vi "FUG_PowerSupply.destructor.vi"(0 "i ref in":refnum<vi>, 5 "error in(no error)":errorcluster) -> (19 "error out":errorcluster)   [LabVIEW 2014, in "FUG_PowerSupply.lvlib"]
doc: "This is the destructor of a class.\n\nLicense Agreement for this software:\n\nCopyright (C)\nGesellschaft für Schwerionenforschung, GSI\nPlanckstr. 1\n64291 Darmstadt\nGermany\n\nContact: D.Beck@gsi.de \n\nThis program is free software; you can redistribute it and/or modify it under the terms of the \nGNU General Public License as published by the Free Software Foundation; either version 2 of \nthe license, or (at your option) any later version.\n\nThis program is distributed in the hope that it will be useful, but WITHOUT ANY WARRANTY; \nwithout even the implied warranty of MERCHANTABILITY or FITNESS FOR A PARTICULAR PURPOSE. See the GNU General License for more details (http://www.gnu.org).\n\nGesellschaft für Schwerionenforschung, GSI\nPlanckstr. 1, 64291 Darmstadt, Germany\nFor all questions and ideas contact: M.Richter@gsi.de, H.Brand@gsi.de or D.Beck@gsi.de.\nLast update: 16-JUN-2004"
uses:
  FUG_PowerSupply.lvlib
  CS_Core/CSApplicationBaseClasses/PSChannelBase/PSChannelBase.lvlib
  CSlibraries-extern/DimLVEvent/LVDimInterface/LVDimInterface.lvlib
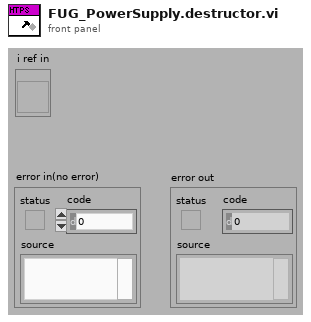
[diagram p1: front panel]
types:
  T1 = typedef "FUG_PowerSupply.lvlib/FUG_PowerSupply.i attribute.ctl" = cluster{"Type":string, "Elektrode Name":string, "CALC_FACTOR_SET_VOLTAGE":dbl, "CALC_FACTOR_GET_VOLTAGE":dbl, "CALC_FACTOR_GET_CURRENT":dbl, "CALC_FACTOR_SET_CURRENT ":dbl, "REG_VALUE":dbl, "Sign":bool, "setVoltID":i32, "setCurrentID":i32, "setPowerOnID":i32, "MaxVoltage":dbl}
  T2 = enum16{"SetAttribute", "GetAttribute", "CreateAttribute", "DestroyAttribute", "DestroyAllAtributes"}
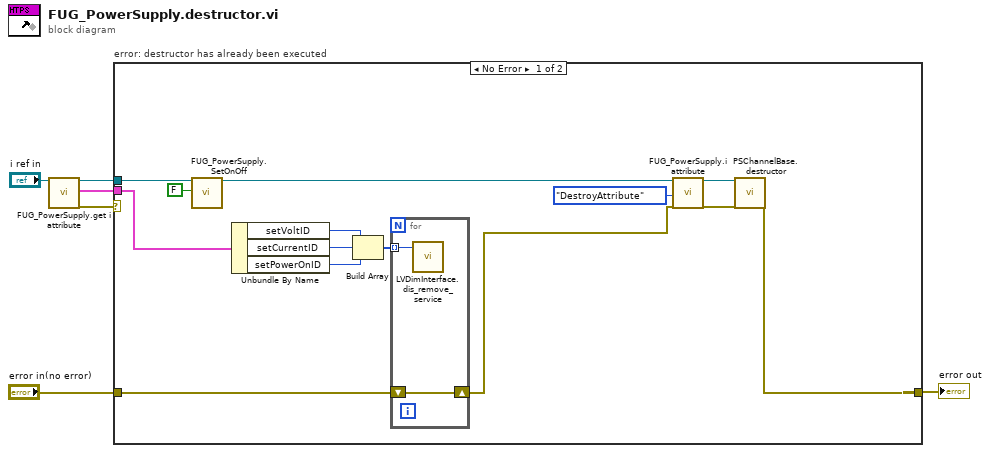
[diagram p0: block diagram]
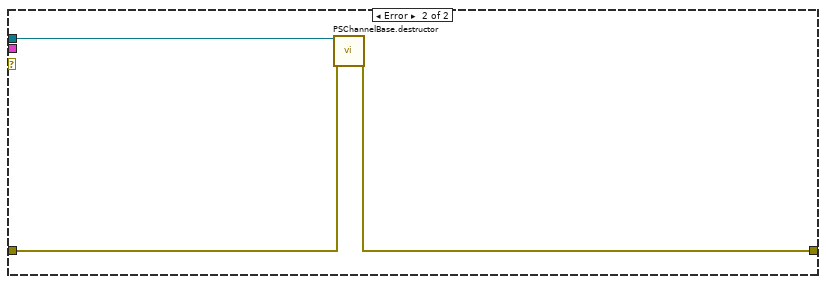
[diagram p2: hidden frame]
diagram:
  n1 = call "FUG_PowerSupply.get i attribute.vi"("i ref in"="i ref in") -> ("i ref out"=w5:refnum<vi>, "i attribute"=w4:T1, "error out"=w3:errorcluster)  [unwired: 16 in]
  n2 = case "error: destructor has already been executed" shown="No Error" w3 {
    tunnel: [w17 w23] -> w1
    tunnel: "error in(no error)" -> [w11 w24]
    tunnel: w5 -> [w9 w25]
    tunnel: w4 -> [w16 _]
    frame No Error {
      n3 = call "FUG_PowerSupply.SetOnOff.vi"("i ref in"=w9, "value"=FALSE) -> ("i ref out"=w8:refnum<vi>)  [unwired: 16 in, 1 out]
      n4 = Unbundle By Name(w16) -> ("setVoltID"=w14:i32, "setCurrentID"=w13:i32, "setPowerOnID"=w15:i32)
      n5 = Build Array(w14, w13, w15) -> (w12:i32[])
      n6 = for {
        tunnel: w12 -> [w22] mode=indexing
        shift-right: [w21] -> w10
        shift-left: w11 -> [w21]
        n7 = call "LVDimInterface.dis_remove_service.vi"("my_serviceID"=w22) -> ()  [unwired: 18 in, 1 out]
      }
      n8 = call "FUG_PowerSupply.i attribute.vi"("VI Refnum"=w8, "Action"=T2."DestroyAttribute", "error in (no error)"=w10) -> ("VI Refnum out"=w19:refnum<vi>, "error out"=w18:errorcluster)  [unwired: 14 in, 1 out]
      n9 = call "PSChannelBase.destructor.vi"("i ref in"=w19, "error in (no error)"=w18) -> ("error out"=w17:errorcluster)  [unwired: 17 in]
    }
    frame Error {
      n10 = call "PSChannelBase.destructor.vi"("i ref in"=w25, "error in (no error)"=w24) -> ("error out"=w23:errorcluster)  [unwired: 17 in]
    }
  }
  "error out" <- w1
